vi "WriteIntakeActuators.vi"(7 "CanGrabStates":T1, 8 "StackClampStates":T2, 9 "Intake Wheel States":T7=enum."Intake Wheels Closed", 10 "Tusk State":T8, 11 "HMI to Control":T3) -> (0 "Stack Clamp Output":bool, 1 "Intake Value":sgl, 2 "Intake Wheel Solenoid Output":bool, 3 "Tusk Solenoid Output":bool, 4 "Can Grab Output":bool, 5 "Wench Value to Control":dbl)   [LabVIEW 2014]
uses:
  Typedefs/TuskStates.ctl
  Typedefs/IntakeWheelStates.ctl
  Typedefs/HMI_to_Control.ctl
  Typedefs/Arm States.ctl
  Typedefs/ClawStates.ctl
  Typedefs/IntakeWheelSenseOrManual.ctl
  Typedefs/StackClampStates.ctl
  Typedefs/Can Grabber.ctl
panel:
  # "Tusks go Down"
  # "Tusks go Up"
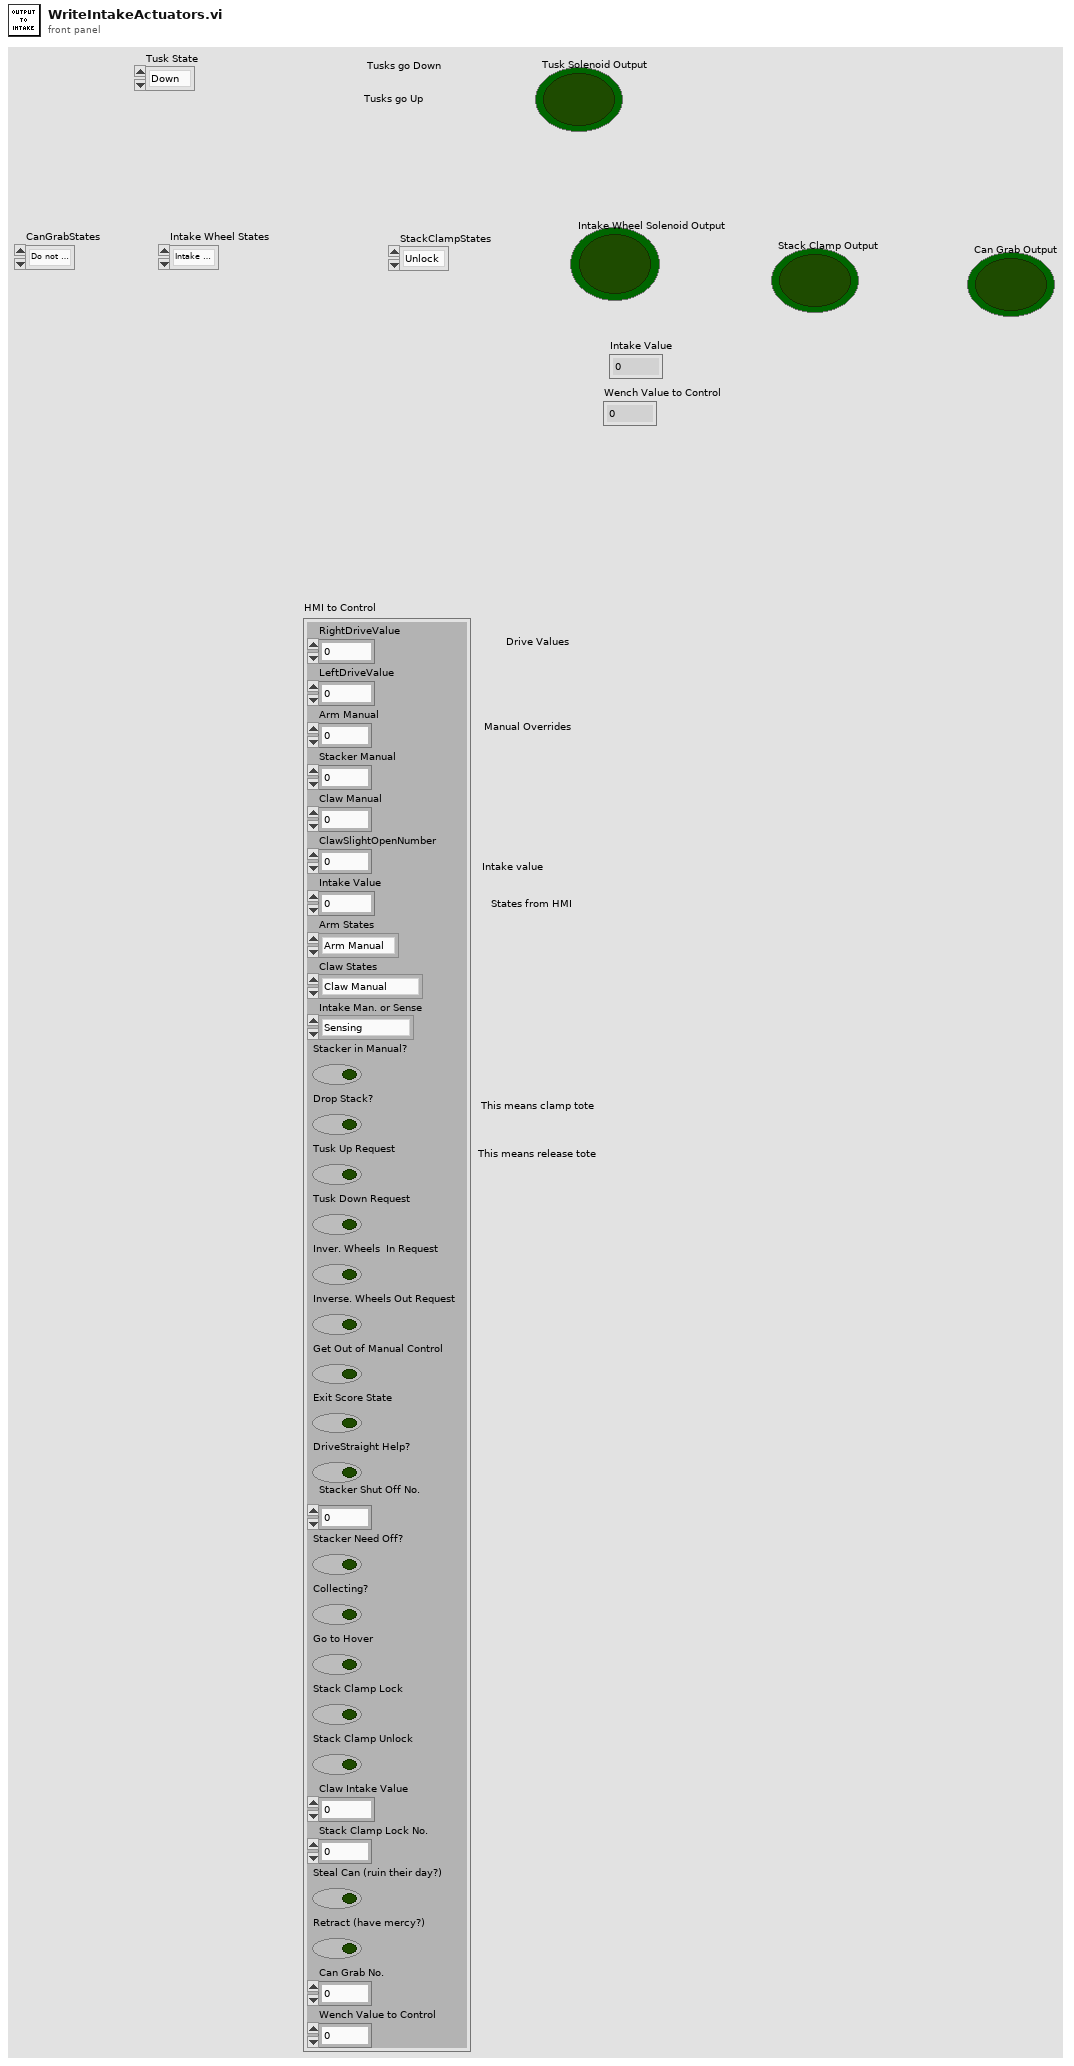
[diagram p1: front panel]
types:
  T1 = typedef "Can Grabber.ctl" = enum16{"Do not steal ", "Steal "}
  T2 = typedef "StackClampStates.ctl" = enum16{"Unlock", "Lock"}
  T3 = typedef "HMI_to_Control.ctl" = cluster{"RightDriveValue":dbl, "LeftDriveValue":dbl, "Arm Manual ":dbl, "Stacker Manual ":dbl, "Claw Manual ":dbl, "ClawSlightOpenNumber":i8, "Intake Value ":sgl, "Arm States":T4, "Claw States":T5, "Intake Man. or Sense":T6, "Stacker in Manual?":bool, "Drop Stack? ":bool, "Tusk Up Request":bool, "Tusk Down Request":bool, "Inver. Wheels  In Request":bool, "Inverse. Wheels Out Request ":bool, "Get Out of Manual Control":bool, "Exit Score State":bool, "DriveStraight Help?":bool, "Stacker Shut Off No.":i8, "Stacker Need Off?":bool, "Collecting?":bool, "Go to Hover":bool, "Stack Clamp Lock ":bool, "Stack Clamp Unlock ":bool, "Claw Intake Value ":sgl, "Stack Clamp Lock No. ":i8, "Steal Can (ruin their day?)":bool, "Retract (have mercy?)":bool, "Can Grab No. ":i8, "Wench Value to Control ":dbl}
  T4 = typedef "Arm States.ctl" = enum16{"Arm Manual ", "Ground", "Step", "1 Tote", "2 Tote", "3 Tote", "4 Tote", "5 Tote", "6 Tote", "Flip Can Arm", "Grab Can in auto", "Nudge"}
  T5 = typedef "ClawStates.ctl" = enum16{"Claw Manual ", "Claw Open", "Claw Closed", "Claw Slight Open", "Flip Can"}
  T6 = typedef "IntakeWheelSenseOrManual.ctl" = enum16{"Sensing", "Manual "}
  T7 = typedef "IntakeWheelStates.ctl" = enum16{"Intake Wheels Open", "Intake Wheels Closed", "Decide off of Input", "Delay before Close", "Operator Request"}
  T8 = typedef "TuskStates.ctl" = enum16{"Down", "Up"}
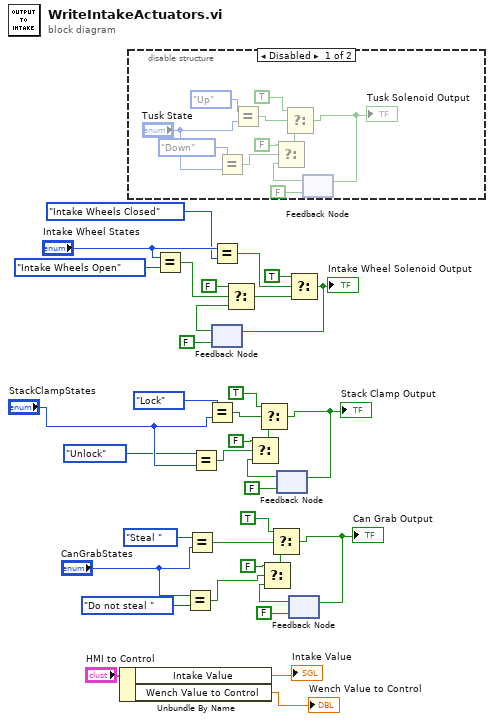
[diagram p0: block diagram]
diagram:
  n1 = Unbundle By Name("HMI to Control") -> ("Intake Value"=→"Intake Value":sgl, "Wench Value to Control"=→"Wench Value to Control":dbl)
  n2 = disable-structure shown="Disabled" {
    frame Disabled {
      n3 = Equal?(x=TuskStates."Down" ("Tusk State 2"), y="Tusk State") -> (x = y?=w42:bool)
      n4 = Equal?(x=TuskStates."Up" ("Tusk State 2"), y="Tusk State") -> (x = y?=w46:bool)
      n5 = feedback #1(FALSE ("Tusk Solenoid Input 2")) -> (w38:bool)
      n6 = Select(t=FALSE ("Tusk Solenoid Input 2"), s=w42, f=w38) -> (s? t:f=w40:bool)
      n7 = Select(t=TRUE ("Tusk Solenoid Input 2"), s=w46, f=w40) -> (s? t:f=w39:bool)
      "Tusk Solenoid Output" <- w39
      n8 = feedback-in #1(w39) -> ()
    }
    frame Enabled {
    }
  }
  n9 = Equal?(x="Intake Wheel States", y=IntakeWheelStates."Intake Wheels Open" ("Intake Wheel States 2")) -> (x = y?=w35:bool)
  n10 = Equal?(x="CanGrabStates", y=Can_Grabber."Do not steal ") -> (x = y?=w2:bool)
  n11 = Equal?(x=Can_Grabber."Steal ", y="CanGrabStates") -> (x = y?=w3:bool)
  n12 = Equal?(x=StackClampStates."Unlock" ("StackClampStates 3"), y="StackClampStates") -> (x = y?=w21:bool)
  n13 = Equal?(x=StackClampStates."Lock" ("StackClampStates 2"), y="StackClampStates") -> (x = y?=w23:bool)
  n14 = Equal?(x="Intake Wheel States", y=IntakeWheelStates."Intake Wheels Closed" ("Intake Wheel States 2")) -> (x = y?=w33:bool)
  n15 = feedback #2(FALSE ("Tusk Solenoid Input 2")) -> (w27:bool)
  n16 = Select(t=FALSE ("Tusk Solenoid Input 2"), s=w35, f=w27) -> (s? t:f=w29:bool)
  n17 = feedback #3(FALSE ("Tusk Solenoid Input 2")) -> (w17:bool)
  n18 = Select(t=FALSE ("Tusk Solenoid Input 2"), s=w21, f=w17) -> (s? t:f=w19:bool)
  n19 = Select(t=TRUE ("Tusk Solenoid Input 2"), s=w23, f=w19) -> (s? t:f=w18:bool)
  "Stack Clamp Output" <- w18
  n20 = feedback-in #3(w18) -> ()
  n21 = Select(t=TRUE ("Tusk Solenoid Input 2"), s=w33, f=w29) -> (s? t:f=w28:bool)
  "Intake Wheel Solenoid Output" <- w28
  n22 = feedback-in #2(w28) -> ()
  n23 = feedback #4(FALSE ("Tusk Solenoid Input 2")) -> (w5:bool)
  n24 = Select(t=FALSE ("Tusk Solenoid Input 2"), s=w2, f=w5) -> (s? t:f=w7:bool)
  n25 = Select(t=TRUE ("Tusk Solenoid Input 2"), s=w3, f=w7) -> (s? t:f=w6:bool)
  "Can Grab Output" <- w6
  n26 = feedback-in #4(w6) -> ()
